vi "AttachHeader.vi"(8 "error in (no error)":errorcluster, 11 "EventFile in":refnum<class "EventFile.lvclass">) -> (0 "error out":errorcluster, 3 "EventFile out":refnum<class "EventFile.lvclass">)   [LabVIEW 2016, in "Event Logging.lvlib" / "EventFile.lvclass"]
uses:
  EventFile.lvclass
  EventFile.lvclass/EventFile.ctl
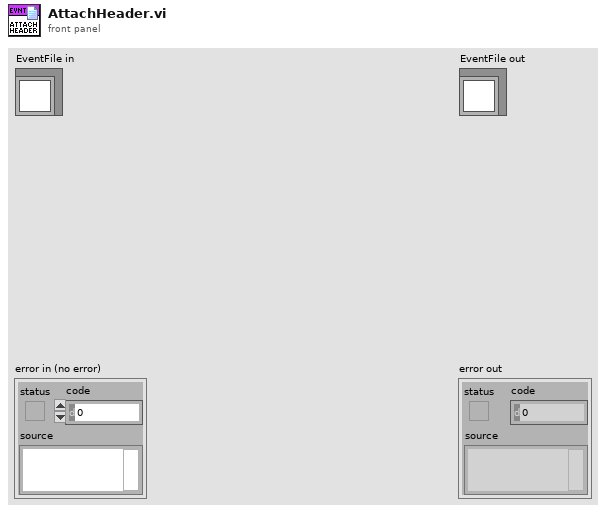
[diagram p1: front panel]
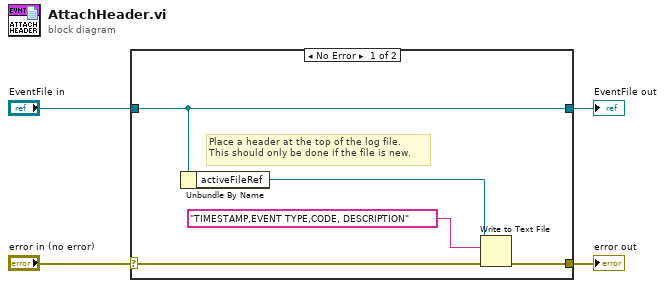
[diagram p0: block diagram]
diagram:
  n1 = case shown="No Error" "error in (no error)" {
    selector: "error in (no error)" -> [w7 w11]
    tunnel: [w6 w11] -> w3
    tunnel: [w9 w10] -> w1
    tunnel: "EventFile in" -> [w9 w10]
    frame No Error {
      # "Place a header at the top of the log file.\nThis should only be done if the file is new."
      n2 = Unbundle By Name(w9) -> ("activeFileRef"=w8:refnum<file>)
      n3 = Write to Text File(file (use dialog)=w8, text="TIMESTAMP,EVENT TYPE,CODE, DESCRIPTION", error in=w7) -> (error out=w6:errorcluster)  [unwired: 1 in, 2 out]
    }
    frame Error {
    }
  }
  "error out" <- w3
  "EventFile out" <- w1
